vi "Set_AIO_Config.vi"(4 "#AnalogOutputs":u16, 6 "#AnalogInputs":u16, 8 "error in (no error)":errorcluster, 9 "StartAddress_AO":u16, 10 "StartAddress_AI":u16, 11 "Device in":refnum<class "DAQ_Device.lvclass">) -> (0 "error out":errorcluster, 3 "Device out":refnum<class "DAQ_Device.lvclass">)   [LabVIEW 2023, in "DAQ_Device.lvclass"]
uses:
  DAQ_Device.lvclass
  DAQ_Device.lvclass/DAQ_Device.ctl
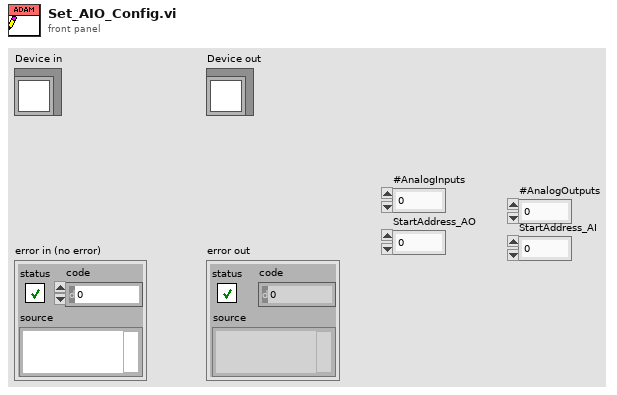
[diagram p1: front panel]
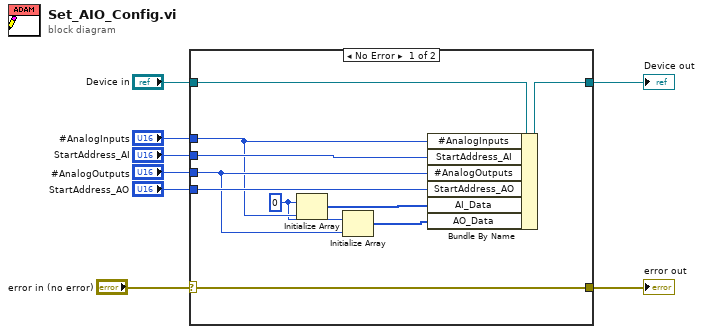
[diagram p0: block diagram]
diagram:
  n1 = case shown="No Error" "error in (no error)" {
    selector: "error in (no error)" -> [w12 w19]
    tunnel: [w12 w19] -> w7
    tunnel: [w17 w20] -> w5
    tunnel: "Device in" -> [w18 w20]
    tunnel: "StartAddress_AO" -> [w16 _]
    tunnel: "StartAddress_AI" -> [w15 _]
    tunnel: "#AnalogOutputs" -> [w14 _]
    tunnel: "#AnalogInputs" -> [w13 _]
    frame No Error {
      w9 = u16 0
      n2 = Initialize Array(w9, w13) -> (w11:u16[])
      n3 = Initialize Array(w9, w14) -> (w10:u16[])
      n4 = Bundle By Name(cluster=w18, "#AnalogInputs"=w13, "StartAddress_AI"=w15, "#AnalogOutputs"=w14, "StartAddress_AO"=w16, "AI_Data"=w11, "AO_Data"=w10) -> (w17:refnum<class "DAQ_Device.lvclass">)
    }
    frame Error {
    }
  }
  "error out" <- w7
  "Device out" <- w5
